vi "Get FFT - Welch PSD.vi"(0 "reference in":refnum<class "GSwFormDSP.lvclass">, 5 "error in (no error)":errorcluster, 6 "Acoustic Weighting":T2, 7 "Spectrum Display Options":T1) -> (13 "Welch PSD":waveform(dbl)[](array[waveform]), 14 "reference out":refnum<class "GSwFormDSP.lvclass">, 19 "error out":errorcluster)   [LabVIEW 2020, in "GSwFormDSP.lvclass"]
uses:
  GSwFormDSP.lvclass
  functions/Acoustic Weighting.ctl
  functions/Spectrum Display Options.ctl
  functions/Spectral Function Type.ctl
  <vilib>/Analysis/_algsub.llb/Vector Norm Type.ctl
  <vilib>/Analysis/_algsub.llb/Real Vector Norm.vi
  <vilib>/Analysis/0measdsp.llb/Scaled Time Domain Window (DBL).vi
  <vilib>/Analysis/NI_AALPro.lvlib
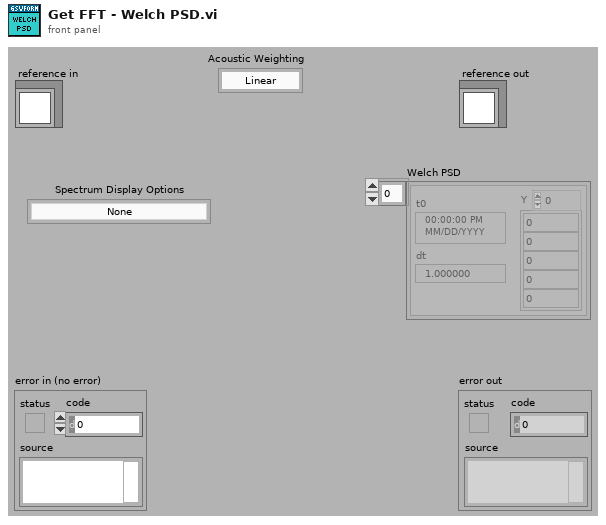
[diagram p1: front panel]
types:
  T1 = typedef "GSwFormDSP.lvclass/Spectrum Display Options.ctl" = enum16{"None", "dB - NO reference value", "dB - Automatic reference value", "dB - Sound SPL (ref 20E-6 Pa)", "dB - Acceleration (ref 1E-6 m/s²)", "dB - Velocity (ref 1E-9 m/s)", "dB - Displacement (ref 1E-12 m)"}
  T2 = typedef "GSwFormDSP.lvclass/Acoustic Weighting.ctl" = enum16{"Linear", "A-weighting"}
  T3 = typedef "GSwFormDSP.lvclass/Spectral Function Type.ctl" = enum16{"Auto Spectrum - (EU RMS)", "Auto Spectrum - (EU Peak)", "Power Spectrum - (EU RMS²)", "Power Spectrum - (EU Peak²)", "Auto Spectrum Density - (EU RMS/rtHz)", "Auto Spectrum Density - (EU Peak/rtHz)", "Power Spectrum Density - (EU RMS²/Hz)", "Power Spectrum Density - (EU Peak²/Hz)"}
  T4 = enum32{"Vrms", "Vpk", "Vrms^2", "Vpk^2", "Vrms/rtHz", "Vpk/rtHz", "Vrms^2/Hz", "Vpk^2/Hz"}
  T5 = enum16{"Power (Vrms^2)", "Amplitude (Vrms)", "Gain (amplitude ratio)"}
  T6 = typedef "GSwFormDSP.lvclass/ObjectAttributes.ctl" = cluster{"Wform Ref":refnum<data-value>, "Nb Signals":i32, "Spectral Function Parameters":T7, "FFT":waveform(cdb)[], "Nb FFT":i32, "Nb Averages":i32[], "Reference Indexes":i32[], "Response Indexes":i32[], "Coherence":waveform(dbl)[], "TDF Parameters":T9, "DAQ":cluster{"Duration (sec)":dbl, "Buffer Size (Samples)":i32, "Offset (Samples)":i32}, "Filter Impulse Response (TDF)":waveform(dbl), "Sound Playback":T10}
  T7 = typedef "GSwFormDSP.lvclass/Spectral Parameters.ctl" = cluster{"Frequency resolution (Hz)":dbl, "Overlap":dbl, "Window":T8}
  T8 = typedef "NI_AALPro.lvlib/windowTd.ctl" = u32
  T9 = typedef "GSwFormDSP.lvclass/TDF Parameters.ctl" = cluster{"Filter":enum32{"Lowpass", "Highpass", "Bandpass", "Bandstop"}, "Type:":enum16{"Butterworth", "Chebyshev", "Inv Chebyshev", "Elliptic", "Bessel"}, "LP cutoff freq":dbl, "HP cutoff freq":dbl, "Order":i32, "passband ripple (dB)":dbl, "stopband attenuation (dB)":dbl, "Phaseless Filter":bool, "Include Fade IN and OUT":bool}
  T10 = typedef "GSwFormDSP.lvclass/Sound Playback.ctl" = cluster{"Timer start (ms)":u32, "task ID":T11, "Cursor Init Location (s)":dbl, "SC Volume":dbl}
  T11 = typedef "Sound Output Task ID.ctl" = u32
  T12 = typedef "NI_AALPro.lvlib/Vector Norm Type.ctl" = u16
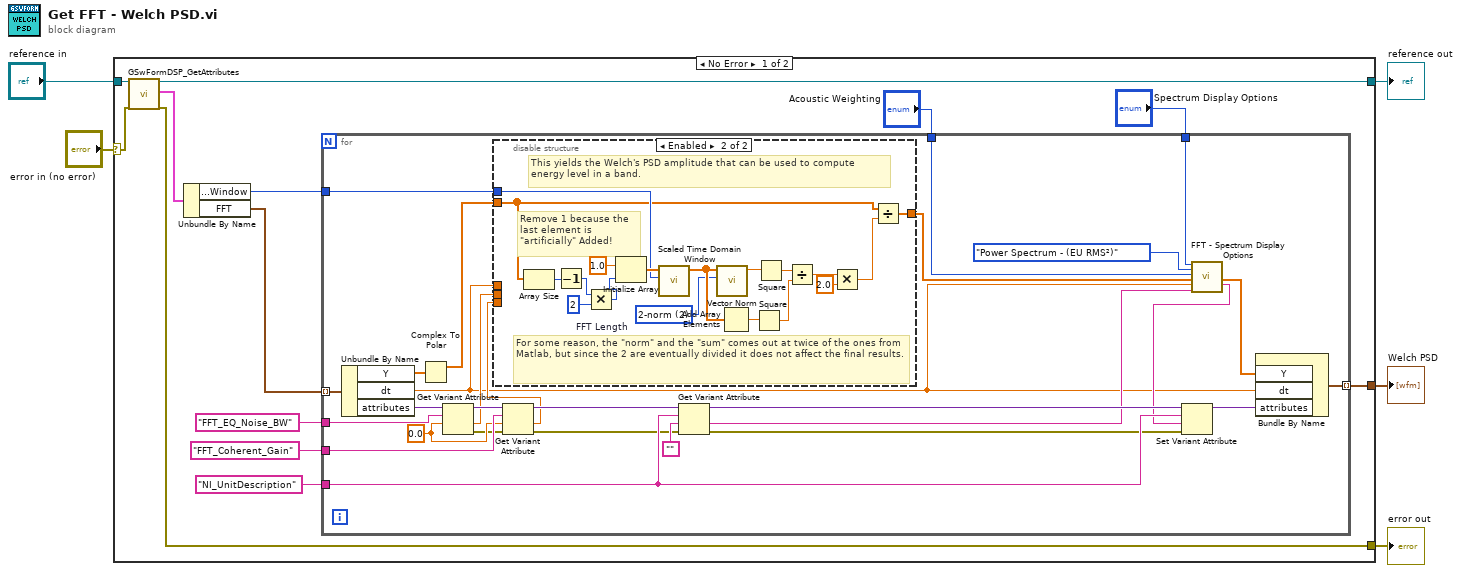
[diagram p0: block diagram]
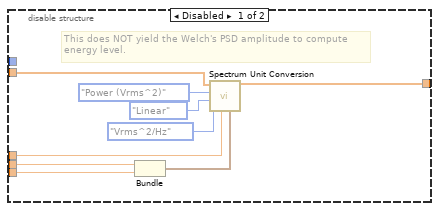
[diagram p2: hidden frame]
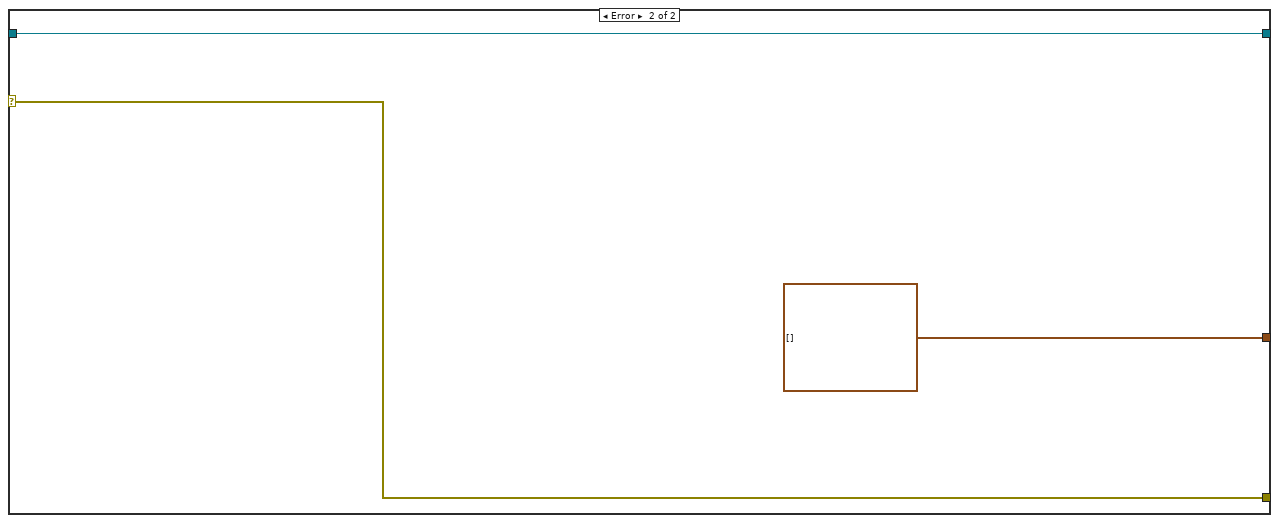
[diagram p3: hidden frame]
diagram:
  n1 = case shown="No Error" "error in (no error)" {
    selector: "error in (no error)" -> [w18 w76]
    tunnel: [w17 w76] -> w4
    tunnel: [w16 w75] -> w2
    tunnel: "reference in" -> [w14 w75]
    tunnel: [w9 waveform(dbl)[] []] -> w1
    frame No Error {
      n2 = call "GSwFormDSP_GetAttributes.vi"("reference in"=w14, "error in (no error)"=w18) -> ("reference out"=w16:refnum<class "GSwFormDSP.lvclass">, "attributes"=w15:T6, "error out"=w17:errorcluster)  [unwired: 14 in, 1 out]
      n3 = Unbundle By Name(w15) -> ("Spectral Function Parameters.Window"=w8:T8, "FFT"=w10:waveform(cdb)[])
      n4 = for {
        tunnel: "FFT_EQ_Noise_BW" ("EQ noise BW (DBL)") -> [w46]
        tunnel: "FFT_Coherent_Gain" ("Coherent Gain (DBL)") -> [w45]
        tunnel: "NI_UnitDescription" ("wform unit") -> [w44]
        tunnel: w10 -> [w43] mode=indexing
        tunnel: [w31] -> w9 mode=indexing
        tunnel: w8 -> [w29]
        tunnel: "Acoustic Weighting" -> [w20]
        tunnel: "Spectrum Display Options" -> [w26]
        w40 = 0.0
        n5 = Unbundle By Name(w43) -> ("Y"=w42:cdb[], "dt"=w19:dbl, "attributes"=w41:variant)
        n6 = Complex To Polar(r * e^(i*theta)=w42) -> (r=w28:dbl[])  [unwired: 1 out]
        n7 = Get Variant Attribute(Variant=w41, name=w46, default value (empty Variant)=w40) -> (duplicate Variant=w39:variant, value=w30:dbl, error out=w38:errorcluster)  [unwired: 1 in, 1 out]
        n8 = Get Variant Attribute(Variant=w39, name=w45, default value (empty Variant)=w40, error in=w38) -> (duplicate Variant=w32:variant, value=w27:dbl, error out=w33:errorcluster)  [unwired: 1 out]
        n9 = disable-structure shown="Enabled" {
          disable-tunnel: w28 -> [w52 w63]
          disable-tunnel: w27 -> [w51 _]
          disable-tunnel: w19 -> [w49 _]
          disable-tunnel: w30 -> [w48 _]
          disable-tunnel: [w47 w62] -> w21
          disable-tunnel: w29 -> [_ w71]
          frame Disabled {
            # "This does NOT yield the Welch's PSD amplitude to compute energy level."
            n10 = Bundle(w48, w51) -> (w53:cluster{dbl, dbl})  [unwired: 1 out]
            n11 = call <vilib>:"Spectrum Unit Conversion.vi"("window constants"=w53, "df"=w49, "display unit"=T4."Vrms^2/Hz", "log/linear"=enum16{"Linear", "dB", "dBm"}."Linear", "spectrum type"=T5."Power (Vrms^2)", "Spectrum in"=w52) -> ("Spectrum out"=w47:dbl[])  [unwired: 1 in, 4 out]
          }
          frame Enabled {
            w60 = T12 2 items=["1-norm"=1, "2-norm"=2, "Inf-norm"=3, "-Inf-norm"=4, "User Defined"=5] ("norm type")
            # "For some reason, the \"norm\" and the \"sum\" comes out at twice of the ones from Matlab, but since the 2 are eventually divided it does not affect the final results."
            # "This yields the Welch's PSD amplitude that can be used to compute energy level in a band."
            # "Remove 1 because the last element is \"artificially\" Added!"
            n12 = Array Size(array=w63) -> (size(s)=w73:i32)
            n13 = Decrement(x=w73) -> (x-1=w58:i32)
            n14 = Multiply "FFT Length"(x=w58, y=2) -> (x*y=w56:i32)
            n15 = Initialize Array(1.0 ("element"), w56) -> (w72:dbl[])
            n16 = call-poly <vilib>:"Scaled Time Domain Window.vi"("window"=w71, "X"=w72) -> ("Windowed X"=w68:dbl[])  [unwired: 1 in, 8 out]
            n17 = call-poly <vilib>:"Vector Norm.vi"("norm type"=w60, "Input Vector"=w68) -> ("norm"=w70:dbl)  [unwired: 8 in, 1 out]
            n18 = Add Array Elements(numeric array=w68) -> (sum=w67:dbl)
            n19 = Square(x=w67) -> (x^2=w66:dbl)
            n20 = Square(x=w70) -> (x^2=w69:dbl)
            n21 = Divide(x=w69, y=w66) -> (x/y=w65:dbl)
            n22 = Multiply(x=w65, y=2.0) -> (x*y=w61:dbl)
            n23 = Divide(x=w63, y=w61) -> (x/y=w62:dbl[])
          }
        }
        n24 = Get Variant Attribute(Variant=w32, name=w44, default value (empty Variant)="", error in=w33) -> (duplicate Variant=w35:variant, value=w22:string, error out=w34:errorcluster)  [unwired: 1 out]
        n25 = call "FFT - Spectrum Display Options.vi"("Spectrum Display Options"=w26, "Spectral Function Type"=Spectral_Function_Type."Power Spectrum - (EU RMS²)", "Acoustic Weighting"=w20, "Spectrum Mag IN"=w21, "dF (Hz)"=w19, "Unit IN"=w22) -> ("Spectrum Mag OUT"=w24:dbl[], "Unit OUT"=w25:string)  [unwired: 12 in]
        n26 = Set Variant Attribute(Variant=w35, name=w44, value=w25, error in=w34) -> (Variant out=w36:variant)  [unwired: 2 out]
        n27 = Bundle By Name("Y"=w24, "dt"=w19, "attributes"=w36) -> (w31:waveform(dbl))  [unwired: 1 in]
      }
    }
    frame Error {
    }
  }
  "error out" <- w4
  "reference out" <- w2
  "Welch PSD" <- w1
